vi "Fill Tree.vi"(8 "Error In":errorcluster, 9 "Nest Data":string[][](array[string]), 10 "Tree Ref":refnum<vi>, 11 "Nest Config":T1) -> (0 "Error Out":errorcluster, 2 "Tree Ref":refnum<vi>, 3 "Nest Config":T1)   [LabVIEW 2013, in "LVH-Nest.lvlib"]
uses:
  LVH-Nest.lvlib
  Type Defs/Nest Config.ctl
  <vilib>/httpClient/ClientHandle.ctl
  Type Defs/Session Data.ctl
  <vilib>/httpClient/LabVIEWHTTPClient.lvlib
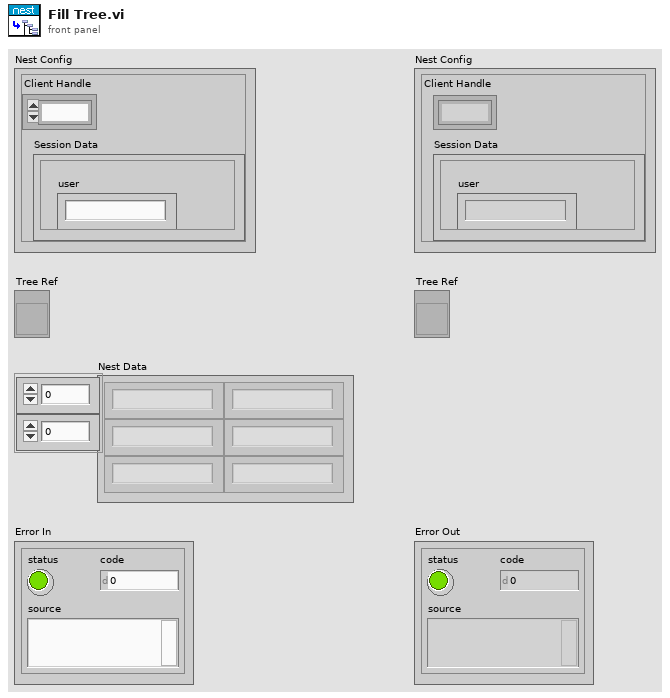
[diagram p1: front panel]
types:
  T1 = typedef "LVH-Nest.lvlib/Nest Config.ctl" = cluster{"Client Handle":T2, "Session Data":T3}
  T2 = typedef "LabVIEWHTTPClient.lvlib/ClientHandle.ctl" = refnum<k1>
  T3 = typedef "LVH-Nest.lvlib/Session Data.ctl" = cluster{"is_superuser":bool, "is_staff":bool, "urls":cluster{"transport_url":string, "rubyapi_url":string, "weather_url":string, "log_upload_url":string, "support_url":string}, "limits":cluster{"thermostats_per_structure":u32, "structures":u32, "thermostats":u32, "smoke_detectors":u32, "smoke_detectors_per_structure":u32}, "access_token":string, "userid":string, "expires_in":string, "email":string, "user":string, "language":string}
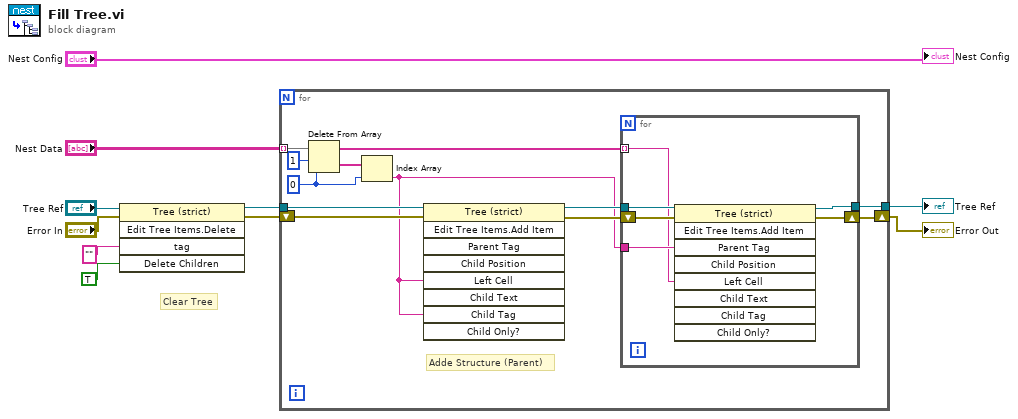
[diagram p0: block diagram]
diagram:
  # "Clear Tree"
  n1 = invoke class="Tree (strict)" method="Edit Tree Items.Delete"(reference="Tree Ref", error in="Error In", "tag"="" ("Tag"), "Delete Children"=TRUE ("Delete Children?")) -> (reference out=w8:refnum<vi>, error out=w7:errorcluster)  [unwired: 1 in, 3 out]
  n2 = for {
    tunnel: w8 -> [w22]
    tunnel: "Nest Data" -> [w20] mode=indexing
    shift-right: [w14] -> w2
    shift-left: w7 -> [w21]
    tunnel: [w11] -> w5
    w17 = 0 ("index")
    # "Adde Structure (Parent)"
    n3 = Delete From Array(array=w20, length=1, index=w17) -> (deleted portion=w18:string[], array with subset deleted=w12:string[])
    n4 = Index Array(array=w18, index=w17) -> (element=w13:string)
    n5 = invoke class="Tree (strict)" method="Edit Tree Items.Add Item"(reference=w22, error in=w21, "Left Cell"=w13, "Child Tag"=w13) -> (reference out=w16:refnum<vi>, error out=w15:errorcluster)  [unwired: 5 in, 7 out]
    n6 = for {
      tunnel: w16 -> [w28]
      shift-right: [w26] -> w14
      shift-left: w15 -> [w27]
      tunnel: w13 -> [w25]
      tunnel: w12 -> [w24] mode=indexing
      tunnel: [w23] -> w11
      n7 = invoke class="Tree (strict)" method="Edit Tree Items.Add Item"(reference=w28, error in=w27, "Parent Tag"=w25, "Left Cell"=w24) -> (reference out=w23:refnum<vi>, error out=w26:errorcluster)  [unwired: 5 in, 7 out]
    }
  }
  "Tree Ref" <- w5
  "Error Out" <- w2
  "Nest Config" <- "Nest Config"
